vi "Read Discrete State.vi"(8 "error in":errorcluster, 10 "Channel Name":string, 11 "DAQ970 in":refnum<class "DAQ970.lvclass">) -> (0 "error out":errorcluster, 2 "State":bool, 3 "DAQ970 out":refnum<class "DAQ970.lvclass">)   [LabVIEW 2019, in "DAQ970.lvlib" / "DAQ970.lvclass"]
uses:
  Library/DAQ970.lvclass
  C:/Users/Public/Documents/Development/builds/Instruments/Instruments.lvlibp/Library/Instruments.lvclass
  builds/Instruments/Instruments.lvlibp/Accessors/Read Measured.vi
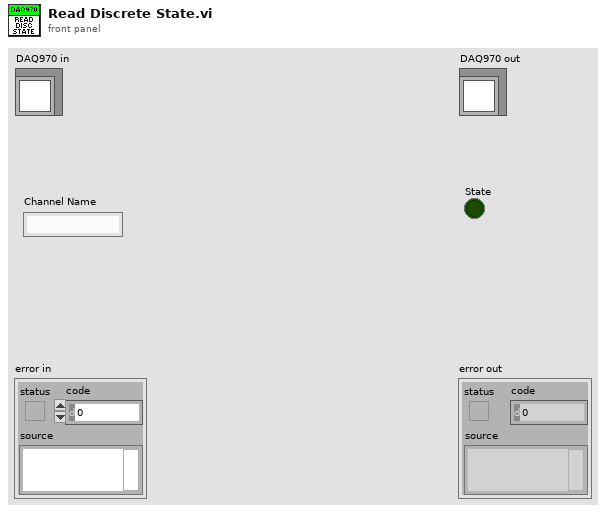
[diagram p1: front panel]
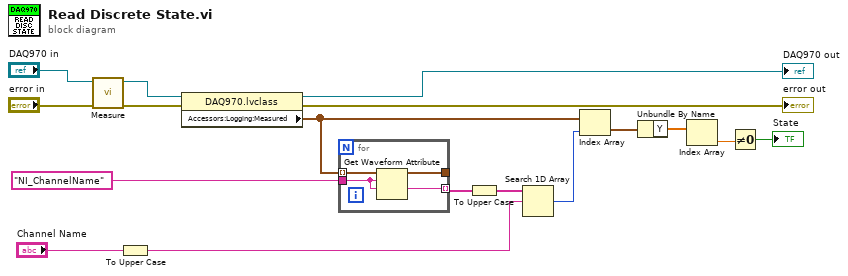
[diagram p0: block diagram]
diagram:
  n1 = call-dynamic "Measure.vi"("error in"="error in", "DAQ970 in"="DAQ970 in") -> ("error out"=w14:errorcluster, "DAQ970 out"=w15:refnum<class "DAQ970.lvclass">)  [unwired: 8 in]
  n2 = To Upper Case(1:"Channel Name") -> (0:w7:string)
  n3 = property class="DAQ970.lvclass"(reference=w15, error in=w14) -> (reference out=→"DAQ970 out":refnum<class "DAQ970.lvclass">, error out=→"error out":errorcluster, "Accessors:Logging:Measured"=w6:waveform(dbl)[])
  n4 = for {
    tunnel: w6 -> [w21] mode=indexing
    tunnel: "NI_ChannelName" ("String") -> [w19]
    tunnel: [w20] -> _
    tunnel: [w18] -> w9 mode=indexing
    n5 = Get Waveform Attribute(5:w19, 6:w19, 7:w21) -> (1:w18:string, 3:w20:waveform(dbl))  [unwired: 1 in, 2 out]
  }
  n6 = To Upper Case(1:w9) -> (0:w8:string[])
  n7 = Search 1D Array(1D array=w8, element=w7) -> (index of element=w5:i32)  [unwired: 1 in]
  n8 = Index Array(array=w6, index=w5) -> (element=w4:waveform(dbl))
  n9 = Unbundle By Name(w4) -> ("Y"=w3:dbl[])
  n10 = Index Array(array=w3) -> (element=w2:dbl)  [unwired: 1 in]
  n11 = Not Equal To 0?(x=w2) -> (x != 0?=→"State":bool)
